vi "RT_check_health.vi"(8 "error in":errorcluster, 9 "FIFO?":bool, 10 "CPU?":bool, 11 "Memory?":bool) -> (0 "error out":errorcluster, 1 "FIFO":T1, 2 "CPU":T2, 3 "Memory":T3)   [LabVIEW 2020]
uses:
  RT_FIFO_Health.ctl
  RT_CPU_load.ctl
  RT_only_FIFO_Health.ctl
  <resource>/objmgr/nisysapi.rc
  <vilib>/NI_Real-Time Target Support.lvlib
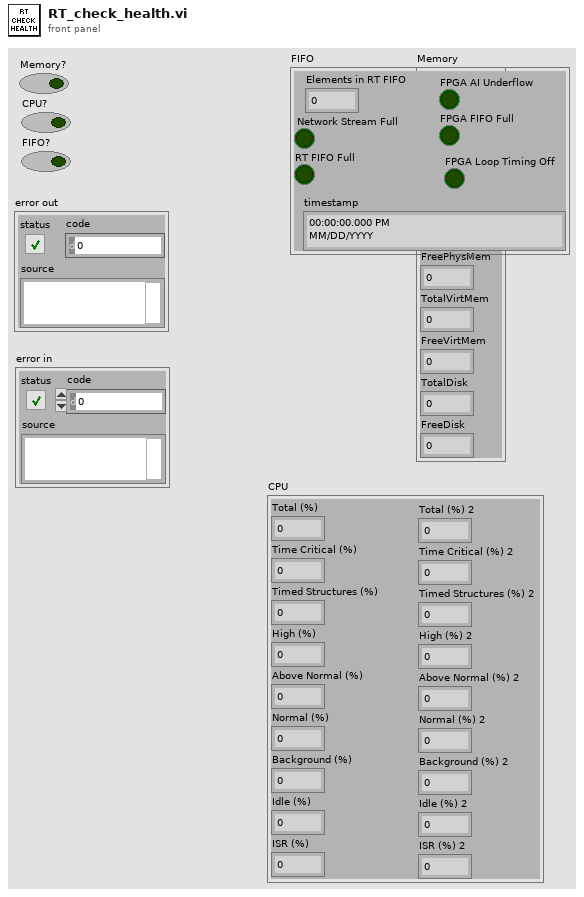
[diagram p1: front panel]
types:
  T1 = typedef "RT_only_FIFO_Health.ctl" = cluster{"Elements in RT FIFO":i32, "Network Stream Full":bool, "RT FIFO Full":bool, "FPGA AI Underflow":bool, "FPGA FIFO Full":bool, "FPGA Loop Timing Off":bool, "timestamp":timestamp}
  T2 = typedef "RT_CPU_load.ctl" = cluster{"Total (%)":dbl, "Time Critical (%)":dbl, "Timed Structures (%)":dbl, "High (%)":dbl, "Above Normal (%)":dbl, "Normal (%)":dbl, "Background (%)":dbl, "Idle (%)":dbl, "ISR (%)":dbl, "ISR (%) 2":dbl, "Idle (%) 2":dbl, "Background (%) 2":dbl, "Normal (%) 2":dbl, "Above Normal (%) 2":dbl, "High (%) 2":dbl, "Timed Structures (%) 2":dbl, "Time Critical (%) 2":dbl, "Total (%) 2":dbl}
  T3 = typedef "RT_FIFO_Health.ctl" = cluster{dbl, dbl, dbl, "TotalPhysMem":dbl, "FreePhysMem":dbl, "TotalVirtMem":dbl, "FreeVirtMem":dbl, "TotalDisk":dbl, "FreeDisk":dbl}
  T4 = typedef "NI_Real-Time Target Support.lvlib/RT CPU Load.ctl" = cluster{"Total (%)":dbl, "Time Critical (%)":dbl, "Timed Structures (%)":dbl, "High (%)":dbl, "Above Normal (%)":dbl, "Normal (%)":dbl, "Background (%)":dbl, "Idle (%)":dbl, "ISR (%)":dbl}
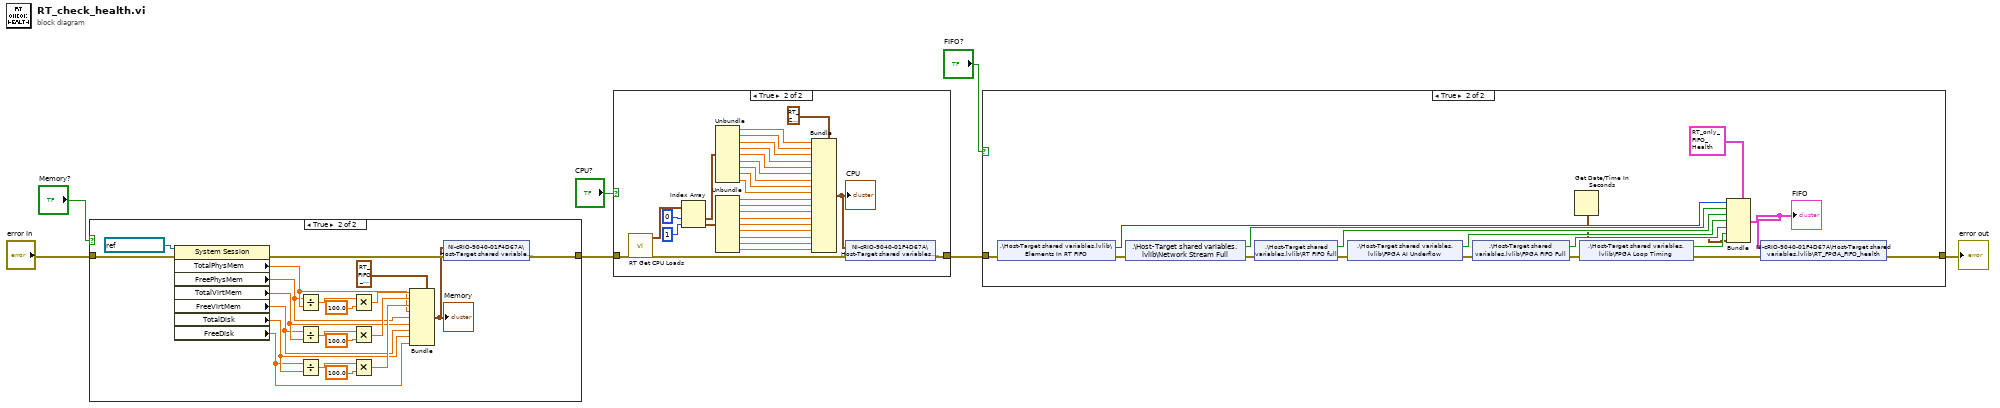
[diagram p0: block diagram]
diagram:
  n1 = case shown="True" "Memory?" {
    tunnel: "error in" -> [w8 w14]
    tunnel: [w8 w9] -> w6
    frame False {
    }
    frame True {
      n2 = property class="System Session"(reference=refnum<k21> "localhost" ("System Session"), error in=w14) -> (error out=w11:errorcluster, "TotalPhysMem"=w16:dbl, "FreePhysMem"=w15:dbl, "TotalVirtMem"=w23:dbl, "FreeVirtMem"=w22:dbl, "TotalDisk"=w27:dbl, "FreeDisk"=w26:dbl)  [unwired: 1 out]
      n3 = Divide(x=w15, y=w16) -> (x/y=w17:dbl)
      n4 = Divide(x=w22, y=w23) -> (x/y=w21:dbl)
      n5 = Divide(x=w26, y=w27) -> (x/y=w25:dbl)
      n6 = Multiply(x=w17, y=100.0) -> (x*y=w19:dbl)
      n7 = Multiply(x=w21, y=100.0) -> (x*y=w24:dbl)
      n8 = Multiply(x=w25, y=100.0) -> (x*y=w28:dbl)
      n9 = Bundle(cluster=T3 {0.0, 0.0, 0.0, "TotalPhysMem"=0.0, "FreePhysMem"=0.0, "TotalVirtMem"=0.0, "FreeVirtMem"=0.0, "TotalDisk"=0.0, "FreeDisk"=0.0} ("output cluster 3"), w19, w24, w28, "TotalPhysMem"=w16, "FreePhysMem"=w15, "TotalVirtMem"=w23, "FreeVirtMem"=w22, "TotalDisk"=w27, "FreeDisk"=w26) -> (w10:T3)
      "Memory" <- w10
      n10 = shared-variable "NI-cRIO-9040-01F4D67A\\Host-Target shared variables.lvlib\\RT_Memory"(w10, error in=w11) -> (error out=w9:errorcluster)
    }
  }
  n11 = case shown="True" "CPU?" {
    tunnel: w6 -> [w30 w34]
    tunnel: [w30 w32] -> w4
    frame False {
    }
    frame True {
      n12 = call <vilib>:"RT Get CPU Loads.vi"("error in (no error)"=w34) -> ("error out"=w33:errorcluster, "CPU loads"=w56:T4[])  [unwired: 9 in]
      n13 = Index Array(array=w56, index #1=0 ("index"), index #2=1 ("index")) -> (element #1=w55:T4, element #2=w45:T4)
      n14 = Unbundle(w55) -> ("Total (%)"=w54:dbl, "Time Critical (%)"=w53:dbl, "Timed Structures (%)"=w52:dbl, "High (%)"=w51:dbl, "Above Normal (%)"=w50:dbl, "Normal (%)"=w49:dbl, "Background (%)"=w48:dbl, "Idle (%)"=w47:dbl, "ISR (%)"=w46:dbl)
      n15 = Unbundle(w45) -> ("Total (%)"=w44:dbl, "Time Critical (%)"=w43:dbl, "Timed Structures (%)"=w42:dbl, "High (%)"=w41:dbl, "Above Normal (%)"=w40:dbl, "Normal (%)"=w39:dbl, "Background (%)"=w38:dbl, "Idle (%)"=w37:dbl, "ISR (%)"=w36:dbl)
      n16 = Bundle(cluster=T2 {"Total (%)"=0.0, "Time Critical (%)"=0.0, "Timed Structures (%)"=0.0, "High (%)"=0.0, "Above Normal (%)"=0.0, "Normal (%)"=0.0, "Background (%)"=0.0, "Idle (%)"=0.0, "ISR (%)"=0.0, "ISR (%) 2"=0.0, "Idle (%) 2"=0.0, "Background (%) 2"=0.0, "Normal (%) 2"=0.0, "Above Normal (%) 2"=0.0, "High (%) 2"=0.0, "Timed Structures (%) 2"=0.0, "Time Critical (%) 2"=0.0, "Total (%) 2"=0.0} ("CPU  2"), "Total (%)"=w54, "Time Critical (%)"=w53, "Timed Structures (%)"=w52, "High (%)"=w51, "Above Normal (%)"=w50, "Normal (%)"=w49, "Background (%)"=w48, "Idle (%)"=w47, "ISR (%)"=w46, "ISR (%) 2"=w44, "Idle (%) 2"=w43, "Background (%) 2"=w42, "Normal (%) 2"=w41, "Above Normal (%) 2"=w40, "High (%) 2"=w39, "Timed Structures (%) 2"=w38, "Time Critical (%) 2"=w37, "Total (%) 2"=w36) -> (w31:T2)
      "CPU" <- w31
      n17 = shared-variable "NI-cRIO-9040-01F4D67A\\Host-Target shared variables.lvlib\\RT CPU Load"(w31, error in=w33) -> (error out=w32:errorcluster)
    }
  }
  n18 = case shown="True" "FIFO?" {
    tunnel: w4 -> [w59 w64]
    tunnel: [w59 w63] -> w2
    frame False {
    }
    frame True {
      n19 = shared-variable ".\\Host-Target shared variables.lvlib\\Elements In RT FIFO"(error in=w64) -> (w74:i32, error out=w73:errorcluster)
      n20 = shared-variable ".\\Host-Target shared variables.lvlib\\Network Stream Full"(error in=w73) -> (w75:bool, error out=w72:errorcluster)
      n21 = shared-variable ".\\Host-Target shared variables.lvlib\\RT FIFO full"(error in=w72) -> (w76:bool, error out=w71:errorcluster)
      n22 = shared-variable ".\\Host-Target shared variables.lvlib\\FPGA AI Underflow"(error in=w71) -> (w68:bool, error out=w70:errorcluster)
      n23 = shared-variable ".\\Host-Target shared variables.lvlib\\FPGA FIFO Full"(error in=w70) -> (w67:bool, error out=w69:errorcluster)
      n24 = Get Date/Time In Seconds() -> (seconds since 1Jan1904=w62:timestamp)
      n25 = shared-variable ".\\Host-Target shared variables.lvlib\\FPGA Loop Timing"(error in=w69) -> (w66:bool, error out=w65:errorcluster)
      n26 = Bundle(cluster=T1 {"Elements in RT FIFO"=0, "Network Stream Full"=FALSE, "RT FIFO Full"=FALSE, "FPGA AI Underflow"=FALSE, "FPGA FIFO Full"=FALSE, "FPGA Loop Timing Off"=FALSE, "timestamp"=timestamp(0 s since 1904-01-01)} ("FIFO 2"), "Elements in RT FIFO"=w74, "Network Stream Full"=w75, "RT FIFO Full"=w76, "FPGA AI Underflow"=w68, "FPGA FIFO Full"=w67, "FPGA Loop Timing Off"=w66, "timestamp"=w62) -> (w60:T1)
      "FIFO" <- w60
      n27 = shared-variable "NI-cRIO-9040-01F4D67A\\Host-Target shared variables.lvlib\\RT_FPGA_FIFO_health"(w60, error in=w65) -> (error out=w63:errorcluster)
    }
  }
  "error out" <- w2
